vi "CLD 10 CSV file utility.vi"(8 "Fehler (Eingang)":T1, 10 "[Daten, Eingang]":T2[](array[typedef]), 11 "CSV-Datei-Enum":T3) -> (0 "Fehler (Ausgang)":T1, 3 "[Daten, Ausgang]":T2[](array[typedef]))   [LabVIEW 2009]
doc: "Dieses VI ist eine funktionale globale Variable (FGV) zum Auslesen der Datei \"CLD CSV File.csv\" und Einfügen der Daten in den Daten-Cluster \"CLD 10 CSV file data structure.ctl\".\n\nHinweis für das Testen:\n\nEs ist ein boolesches Element vorhanden, mit dem sichergestellt werden kann, dass die FGV entweder im gleichen Verzeichnis, in dem sich auch die FGV befindet (nützlich für das Testen), oder im Verzeichnis des Aufrufers nach der Datendatei sucht, wenn sich der Aufrufer in einer Standard-CLD-Testhierarchie eine Verzeichnisebene über dem SubVI-Verzeichnis befindet."
uses:
  <vilib>/Utility/file.llb/Read From Spreadsheet File (string).vi
  CLD 10 CSV file data structure.ctl
  <vilib>/Utility/file.llb/Write To Spreadsheet File (string).vi
  CLD 10 CSV file enum.ctl
panel:
  in  "(T) Haupt-VI (F) Sub-VI":bool
  # "Standardeinstellung (T) wird nur für das Testen verwendet"
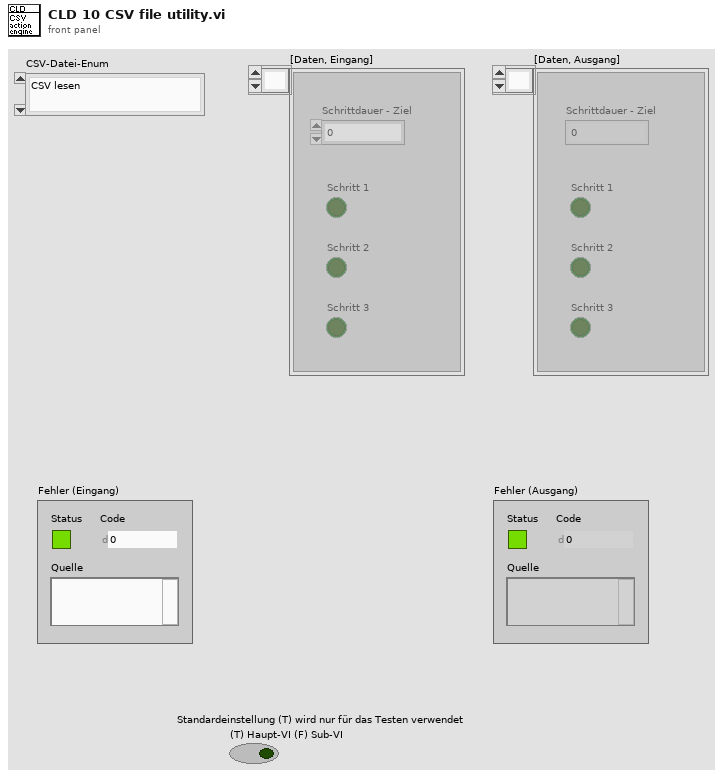
[diagram p1: front panel]
types:
  T1 = cluster{"Status":bool, "Code":i32, "Quelle":string}
  T2 = typedef "CLD 10 CSV file data structure.ctl" = cluster{"Schrittdauer - Ziel":i32, "Schritt 1":bool, "Schritt 2":bool, "Schritt 3":bool}
  T3 = typedef "CLD 10 CSV file enum.ctl" = enum16{"CSV lesen", "CSV schreiben"}
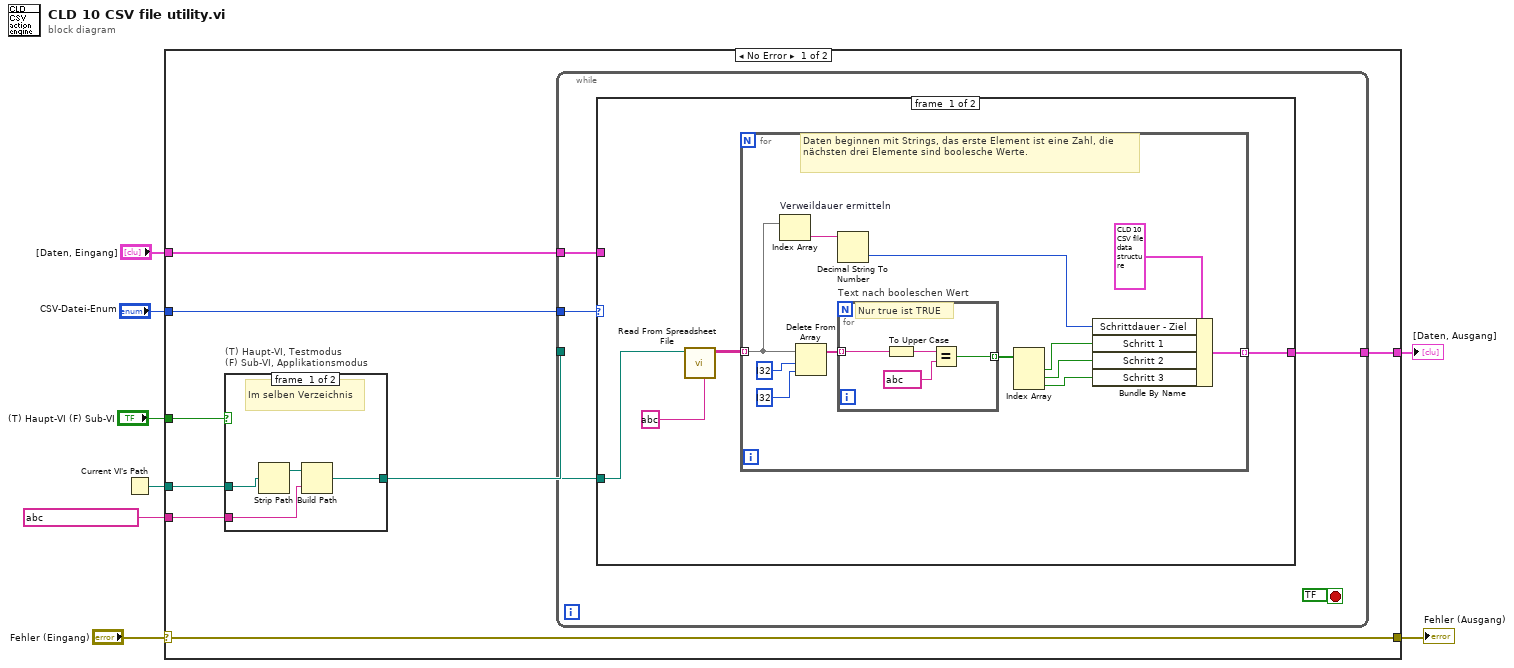
[diagram p0: block diagram]
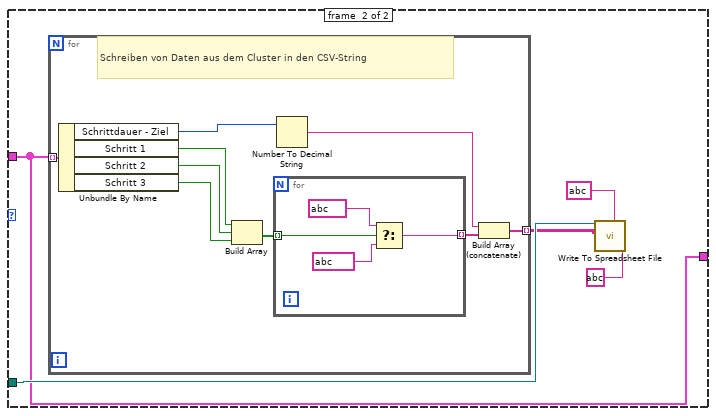
[diagram p2: hidden frame]
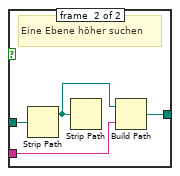
[diagram p3: hidden frame]
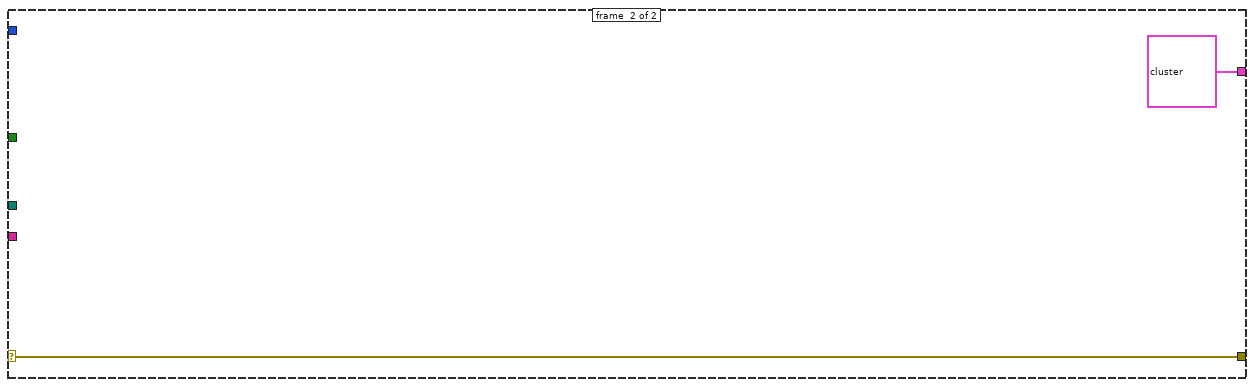
[diagram p4: hidden frame]
diagram:
  n1 = Current VI's Path() -> (path=w5:path)
  n2 = case shown="No Error" "Fehler (Eingang)" {
    selector: "Fehler (Eingang)" -> [w9 w69]
    tunnel: [w16 T2[] ? ("[Daten, Eingang]")] -> w8
    tunnel: "(T) Haupt-VI (F) Sub-VI" -> [w15 _]
    tunnel: string ? -> [w14 _]
    tunnel: w5 -> [w13 _]
    tunnel: "CSV-Datei-Enum" -> [w11 _]
    tunnel: "[Daten, Eingang]" -> [w10 _]
    tunnel: [w9 w69] -> w1
    frame #0 {
      n3 = case "(T) Haupt-VI, Testmodus\n(F) Sub-VI, Applikationsmodus" shown="True" w15 {
        tunnel: w14 -> [w61 w66]
        tunnel: w13 -> [w62 w67]
        tunnel: [w60 w65] -> w12
        frame #0 {
          # "Im selben Verzeichnis"
          n4 = Strip Path(path=w62) -> (stripped path=w63:path)  [unwired: 1 out]
          n5 = Build Path(base path=w63, name or relative path=w61) -> (appended path=w60:path)
        }
        frame #1 {
          # "Eine Ebene höher suchen"
          n6 = Strip Path(path=w67) -> (stripped path=w64:path)  [unwired: 1 out]
          n7 = Strip Path(path=w64) -> ()  [unwired: 2 out]
          n8 = Build Path(base path=w64, name or relative path=w66) -> (appended path=w65:path)
        }
      }
      n9 = while {
        tunnel: w12 -> [w19]
        tunnel: w11 -> [w20]
        tunnel: [w18] -> w16
        tunnel: w10 -> [w17]
        stop <- bool ? stop-if-true
        n10 = case shown="\"CSV schreiben\"" w20 {
          tunnel: w19 -> [w25 w46]
          tunnel: [w23 w42] -> w18
          tunnel: w17 -> [_ w42]
          frame #0 {
            n11 = call-poly <vilib>:"Read From Spreadsheet File.vi"("delimiter (\\t)"=string ? ("Trennzeichen (\\t)"), "file path (dialog if empty)"=w25) -> ("all rows"=w24:string[][])  [unwired: 5 in, 4 out]
            n12 = for {
              tunnel: w24 -> [w34] mode=indexing
              tunnel: [w37] -> w23 mode=indexing
              # "Daten beginnen mit Strings, das erste Element ist eine Zahl, die nächsten drei Elemente sind boolesche Werte."
              n13 = Index Array "Verweildauer ermitteln"(array=w34) -> (element=w36:string)  [unwired: 1 in]
              n14 = Delete From Array(array=w34, length=i32 ? ("Länge"), index=i32 ? ("Index")) -> (array with subset deleted=w27:string[])  [unwired: 1 out]
              n15 = Decimal String To Number(string=w36) -> (number=w35:i32)  [unwired: 2 in, 1 out]
              n16 = for "Text nach booleschen Wert" {
                tunnel: w27 -> [w41] mode=indexing
                tunnel: [w38] -> w31 mode=indexing
                # "Nur true ist TRUE"
                n17 = To Upper Case(1:w41) -> (0:w40:string)
                n18 = Equal?(x=w40, y=string ?) -> (x = y?=w38:bool)
              }
              n19 = Index Array(array=w31) -> (element #1=w30:bool, element #2=w29:bool, element #3=w28:bool)  [unwired: 3 in]
              n20 = Bundle By Name(cluster=T2 ? ("Datenstruktur der CSV-Datei"), "Schrittdauer - Ziel"=w35, "Schritt 1"=w30, "Schritt 2"=w29, "Schritt 3"=w28) -> (w37:T2)
            }
          }
          frame #1 {
            n21 = for {
              tunnel: w42 -> [w55] mode=indexing
              tunnel: [w47] -> w44 mode=indexing
              # "Schreiben von Daten aus dem Cluster in den CSV-String"
              n22 = Unbundle By Name(w55) -> ("Schrittdauer - Ziel"=w54:i32, "Schritt 1"=w53:bool, "Schritt 2"=w52:bool, "Schritt 3"=w51:bool)
              n23 = Build Array(w53, w52, w51) -> (w50:bool[])
              n24 = for {
                tunnel: w50 -> [w59] mode=indexing
                tunnel: [w56] -> w48 mode=indexing
                n25 = Select(t=string ?, s=w59, f=string ?) -> (s? t:f=w56:string)
              }
              n26 = Number To Decimal String(number=w54) -> (decimal integer string=w49:string)  [unwired: 1 in]
              n27 = Build Array (concatenate)(w49, w48) -> (w47:string[])
            }
            n28 = call-poly <vilib>:"Write To Spreadsheet File.vi"("delimiter (\\t)"=string ? ("Trennzeichen (\\t)"), "format (%s)"=string ? ("Format (%s)"), "2D data"=w44, "file path (dialog if empty)"=w46) -> ()  [unwired: 4 in, 1 out]
          }
        }
      }
    }
    frame #1 {
    }
  }
  "[Daten, Ausgang]" <- w8
  "Fehler (Ausgang)" <- w1
